vi "S4GUI.vi"() -> ()   [LabVIEW 2018] (continued)
            n2040 = call-dynamic "Write Suffix.vi"("error in (no error)"=w4728, "Suffix"=w4747, "Interface in"=w4729) -> ("error out"=w4746:errorcluster, "Interface out"=w4740:refnum<class "Interface.lvclass">)  [unwired: 7 in]
            n2041 = call-dynamic "Write ObsType.vi"("error in (no error)"=w4746, "ObsType"=w4732, "Interface in"=w4740) -> ("error out"=w4745:errorcluster, "Interface out"=w4739:refnum<class "Interface.lvclass">)  [unwired: 7 in]
            n2042 = call-dynamic "Write Object.vi"("error in (no error)"=w4745, "Object"=w4731, "Interface in"=w4739) -> ("error out"=w4744:errorcluster, "Interface out"=w4738:refnum<class "Interface.lvclass">)  [unwired: 7 in]
            n2043 = call-dynamic "Write Comments.vi"("error in (no error)"=w4744, "Comments"=w4733, "Interface in"=w4738) -> ("error out"=w4727:errorcluster, "Interface out"=w4726:refnum<class "Interface.lvclass">)  [unwired: 7 in]
            n2044 = call-dynamic "Write Observer.vi"("error in (no error)"=w4727, "Observer"=w4730, "Interface in"=w4726) -> ("error out"=w4722:errorcluster, "Interface out"=w4721:refnum<class "Interface.lvclass">)  [unwired: 7 in]
            n2045 = call-dynamic "Write Interface.vi"("error in (no error)"=w4722, "Interface.lvclass"=w4721, "Channel in"=w4741) -> ("error out"=w4717:errorcluster, "Channel out"=w4720:refnum<class "Channel.lvclass">)  [unwired: 7 in]
            n2046 = call-dynamic "Read State Machine.vi"("error in (no error)"=w4717, "Device in"=w4720) -> ("error out"=w4725:errorcluster, "State Machine.lvclass"=w4715:refnum<class "State Machine.lvclass">, "Device out"=w4719:refnum<class "Channel.lvclass">)  [unwired: 7 in]
            n2047 = call "Next State.vi"("error in (no error)"=w4725, "New_State"=12, "State Machine in"=w4715) -> ("error out"=w4724:errorcluster, "State Machine out"=w4714:refnum<class "State Machine.lvclass">)  [unwired: 7 in]
            n2048 = call-dynamic "Write State Machine.vi"("error in (no error)"=w4724, "State Machine.lvclass"=w4714, "Device in"=w4719) -> ("error out"=w4716:errorcluster, "Device out"=w4718:refnum<class "Channel.lvclass">)  [unwired: 7 in]
            n2049 = call-dynamic "Write Channel.vi"("error in (no error)"=w4716, "Channel.lvclass"=w4718, "Acquisition in"=w4736) -> ("error out"=w4734:errorcluster, "Acquisition out"=w4735:refnum<class "Acquisition.lvclass">)  [unwired: 7 in]
            n2050 = call-dynamic "Write AcquisitionD.vi"("error in (no error)"=w4734, "Acquisition.lvclass"=w4735, "S4ACS_GUI in"=w4737) -> ("error out"=w4748:errorcluster, "S4ACS_GUI out"=w4749:refnum<class "S4GUI.lvclass">)  [unwired: 7 in]
          }
        }
      }
      event "object suffix", "dflat suffix", "sflat suffix", "dark suffix", "zero suffix", "focus suffix": Value Change {
        # "Remove todos <\\n> e <space> do sufixo:"
        n2051 = event-data() -> ("NewVal"=w4760:string)  [unwired: 1 in, 5 out]
        n2052 = To Lower Case(string=w4760) -> (all lower case string=w4759:string)
        n2053 = call <vilib>:"Trim Whitespace.vi"("string"=w4759) -> ("trimmed string"=w4758:string)  [unwired: 1 in]
        n2054 = Search and Replace String(replace all?=TRUE ("replace all? (F)"), input string=w4758, search string="\n") -> (result string=w4756:string)  [unwired: 5 in, 3 out]
        n2055 = call <vilib>:"Space Constant.vi"() -> ("String"=w4754:string)
        n2056 = Search and Replace String(replace all?=TRUE ("replace all? (F)"), input string=w4756, search string=w4754) -> (result string=w4757:string)  [unwired: 5 in, 3 out]
        n2057 = stacked-sequence {
          seq-local: [w4796 _ _ _] -> [_ w4854 _ _]
          seq-local: [w4795 _ _ _] -> [_ w4853 _ _]
          seq-local: [_ w4852 _ _] -> [_ _ w4897 _]
          seq-local: [_ w4851 _ _] -> [_ _ w4896 _]
          seq-local: [_ _ w4895 _] -> [_ _ _ w4940]
          seq-local: [_ _ w4894 _] -> [_ _ _ w4939]
          tunnel: w4767 -> [w4808 _ _ _]
          tunnel: w4768 -> [w4807 _ _ _]
          tunnel: [_ _ _ w4938] -> w4762
          tunnel: [_ _ _ w4937] -> w4761
          tunnel: w4757 -> [w4794 w4850 w4893 w4936]
          tunnel: w4765 -> [w4793 w4849 w4879 w4922]
          tunnel: w4763 -> [w4792 w4835 w4878 w4921]
          tunnel: w4766 -> [w4791 w4834 w4877 w4920]
          tunnel: w4764 -> [w4790 w4833 w4876 w4919]
          frame #0 {
            # "observer"
            # "comment"
            # "object"
            # "suffix"
            # "obsType"
            n2058 = call-dynamic "Read AcquisitionA.vi"("error in (no error)"=w4808, "S4ACS_GUI in"=w4807) -> ("error out"=w4806:errorcluster, "Acquisition.lvclass"=w4805:refnum<class "Acquisition.lvclass">, "S4ACS_GUI out"=w4800:refnum<class "S4GUI.lvclass">)  [unwired: 7 in]
            n2059 = call-dynamic "Read Channel.vi"("error in (no error)"=w4806, "Acquisition in"=w4805) -> ("error out"=w4770:errorcluster, "Channel.lvclass"=w4773:refnum<class "Channel.lvclass">, "Acquisition out"=w4799:refnum<class "Acquisition.lvclass">)  [unwired: 7 in]
            n2060 = local read "Filter1"() -> (w4771:u8)
            n2061 = call-dynamic "Write Filter.vi"("error in (no error)"=w4770, "Filter"=w4771, "Channel in"=w4773) -> ("error out"=w4769:errorcluster, "Channel out"=w4772:refnum<class "Channel.lvclass">)  [unwired: 7 in]
            n2062 = call-dynamic "Read Interface.vi"("error in (no error)"=w4769, "Channel in"=w4772) -> ("error out"=w4786:errorcluster, "Interface.lvclass"=w4787:refnum<class "Interface.lvclass">, "Channel out"=w4804:refnum<class "Channel.lvclass">)  [unwired: 7 in]
            n2063 = call-dynamic "Write Suffix.vi"("error in (no error)"=w4786, "Suffix"=w4794, "Interface in"=w4787) -> ("error out"=w4811:errorcluster, "Interface out"=w4803:refnum<class "Interface.lvclass">)  [unwired: 7 in]
            n2064 = call-dynamic "Write ObsType.vi"("error in (no error)"=w4811, "ObsType"=w4792, "Interface in"=w4803) -> ("error out"=w4810:errorcluster, "Interface out"=w4802:refnum<class "Interface.lvclass">)  [unwired: 7 in]
            n2065 = call-dynamic "Write Object.vi"("error in (no error)"=w4810, "Object"=w4791, "Interface in"=w4802) -> ("error out"=w4809:errorcluster, "Interface out"=w4801:refnum<class "Interface.lvclass">)  [unwired: 7 in]
            n2066 = call-dynamic "Write Comments.vi"("error in (no error)"=w4809, "Comments"=w4793, "Interface in"=w4801) -> ("error out"=w4789:errorcluster, "Interface out"=w4788:refnum<class "Interface.lvclass">)  [unwired: 7 in]
            n2067 = call-dynamic "Write Observer.vi"("error in (no error)"=w4789, "Observer"=w4790, "Interface in"=w4788) -> ("error out"=w4784:errorcluster, "Interface out"=w4785:refnum<class "Interface.lvclass">)  [unwired: 7 in]
            n2068 = call-dynamic "Write Interface.vi"("error in (no error)"=w4784, "Interface.lvclass"=w4785, "Channel in"=w4804) -> ("error out"=w4780:errorcluster, "Channel out"=w4783:refnum<class "Channel.lvclass">)  [unwired: 7 in]
            n2069 = call-dynamic "Read State Machine.vi"("error in (no error)"=w4780, "Device in"=w4783) -> ("error out"=w4779:errorcluster, "State Machine.lvclass"=w4777:refnum<class "State Machine.lvclass">, "Device out"=w4782:refnum<class "Channel.lvclass">)  [unwired: 7 in]
            n2070 = call "Next State.vi"("error in (no error)"=w4779, "New_State"=12, "State Machine in"=w4777) -> ("error out"=w4778:errorcluster, "State Machine out"=w4776:refnum<class "State Machine.lvclass">)  [unwired: 7 in]
            n2071 = call-dynamic "Write State Machine.vi"("error in (no error)"=w4778, "State Machine.lvclass"=w4776, "Device in"=w4782) -> ("error out"=w4775:errorcluster, "Device out"=w4781:refnum<class "Channel.lvclass">)  [unwired: 7 in]
            n2072 = call-dynamic "Write Channel.vi"("error in (no error)"=w4775, "Channel.lvclass"=w4781, "Acquisition in"=w4799) -> ("error out"=w4797:errorcluster, "Acquisition out"=w4798:refnum<class "Acquisition.lvclass">)  [unwired: 7 in]
            n2073 = call-dynamic "Write AcquisitionA.vi"("error in (no error)"=w4797, "Acquisition.lvclass"=w4798, "S4ACS_GUI in"=w4800) -> ("error out"=w4795:errorcluster, "S4ACS_GUI out"=w4796:refnum<class "S4GUI.lvclass">)  [unwired: 7 in]
          }
          frame #1 {
            # "object"
            # "suffix"
            # "obsType"
            n2074 = call "Read AcquisitionB.vi"("error in (no error)"=w4853, "S4ACS_GUI in"=w4854) -> ("error out"=w4839:errorcluster, "Acquisition.lvclass"=w4840:refnum<class "Acquisition.lvclass">, "S4ACS_GUI out"=w4845:refnum<class "S4GUI.lvclass">)  [unwired: 7 in]
            n2075 = call-dynamic "Read Channel.vi"("error in (no error)"=w4839, "Acquisition in"=w4840) -> ("error out"=w4813:errorcluster, "Channel.lvclass"=w4815:refnum<class "Channel.lvclass">, "Acquisition out"=w4846:refnum<class "Acquisition.lvclass">)  [unwired: 7 in]
            n2076 = local read "Filter2"() -> (w4816:u8)
            n2077 = call-dynamic "Write Filter.vi"("error in (no error)"=w4813, "Filter"=w4816, "Channel in"=w4815) -> ("error out"=w4812:errorcluster, "Channel out"=w4814:refnum<class "Channel.lvclass">)  [unwired: 7 in]
            n2078 = call-dynamic "Read Interface.vi"("error in (no error)"=w4812, "Channel in"=w4814) -> ("error out"=w4827:errorcluster, "Interface.lvclass"=w4828:refnum<class "Interface.lvclass">, "Channel out"=w4841:refnum<class "Channel.lvclass">)  [unwired: 7 in]
            n2079 = call-dynamic "Write Suffix.vi"("error in (no error)"=w4827, "Suffix"=w4850, "Interface in"=w4828) -> ("error out"=w4836:errorcluster, "Interface out"=w4842:refnum<class "Interface.lvclass">)  [unwired: 7 in]
            n2080 = call-dynamic "Write ObsType.vi"("error in (no error)"=w4836, "ObsType"=w4835, "Interface in"=w4842) -> ("error out"=w4837:errorcluster, "Interface out"=w4843:refnum<class "Interface.lvclass">)  [unwired: 7 in]
            n2081 = call-dynamic "Write Object.vi"("error in (no error)"=w4837, "Object"=w4834, "Interface in"=w4843) -> ("error out"=w4838:errorcluster, "Interface out"=w4844:refnum<class "Interface.lvclass">)  [unwired: 7 in]
            n2082 = call-dynamic "Write Comments.vi"("error in (no error)"=w4838, "Comments"=w4849, "Interface in"=w4844) -> ("error out"=w4830:errorcluster, "Interface out"=w4829:refnum<class "Interface.lvclass">)  [unwired: 7 in]
            n2083 = call-dynamic "Write Observer.vi"("error in (no error)"=w4830, "Observer"=w4833, "Interface in"=w4829) -> ("error out"=w4831:errorcluster, "Interface out"=w4832:refnum<class "Interface.lvclass">)  [unwired: 7 in]
            n2084 = call-dynamic "Write Interface.vi"("error in (no error)"=w4831, "Interface.lvclass"=w4832, "Channel in"=w4841) -> ("error out"=w4820:errorcluster, "Channel out"=w4821:refnum<class "Channel.lvclass">)  [unwired: 7 in]
            n2085 = call-dynamic "Read State Machine.vi"("error in (no error)"=w4820, "Device in"=w4821) -> ("error out"=w4826:errorcluster, "State Machine.lvclass"=w4824:refnum<class "State Machine.lvclass">, "Device out"=w4819:refnum<class "Channel.lvclass">)  [unwired: 7 in]
            n2086 = call "Next State.vi"("error in (no error)"=w4826, "New_State"=12, "State Machine in"=w4824) -> ("error out"=w4825:errorcluster, "State Machine out"=w4823:refnum<class "State Machine.lvclass">)  [unwired: 7 in]
            n2087 = call-dynamic "Write State Machine.vi"("error in (no error)"=w4825, "State Machine.lvclass"=w4823, "Device in"=w4819) -> ("error out"=w4817:errorcluster, "Device out"=w4818:refnum<class "Channel.lvclass">)  [unwired: 7 in]
            n2088 = call-dynamic "Write Channel.vi"("error in (no error)"=w4817, "Channel.lvclass"=w4818, "Acquisition in"=w4846) -> ("error out"=w4848:errorcluster, "Acquisition out"=w4847:refnum<class "Acquisition.lvclass">)  [unwired: 7 in]
            n2089 = call "Write AcquisitionB.vi"("error in (no error)"=w4848, "Acquisition.lvclass"=w4847, "S4ACS_GUI in"=w4845) -> ("error out"=w4851:errorcluster, "S4ACS_GUI out"=w4852:refnum<class "S4GUI.lvclass">)  [unwired: 7 in]
          }
          frame #2 {
            # "object"
            # "suffix"
            # "obsType"
            n2090 = call-dynamic "Read AcquisitionC.vi"("error in (no error)"=w4896, "S4ACS_GUI in"=w4897) -> ("error out"=w4889:errorcluster, "Acquisition.lvclass"=w4888:refnum<class "Acquisition.lvclass">, "S4ACS_GUI out"=w4883:refnum<class "S4GUI.lvclass">)  [unwired: 7 in]
            n2091 = call-dynamic "Read Channel.vi"("error in (no error)"=w4889, "Acquisition in"=w4888) -> ("error out"=w4856:errorcluster, "Channel.lvclass"=w4858:refnum<class "Channel.lvclass">, "Acquisition out"=w4882:refnum<class "Acquisition.lvclass">)  [unwired: 7 in]
            n2092 = local read "Filter3"() -> (w4859:u8)
            n2093 = call-dynamic "Write Filter.vi"("error in (no error)"=w4856, "Filter"=w4859, "Channel in"=w4858) -> ("error out"=w4855:errorcluster, "Channel out"=w4857:refnum<class "Channel.lvclass">)  [unwired: 7 in]
            n2094 = call-dynamic "Read Interface.vi"("error in (no error)"=w4855, "Channel in"=w4857) -> ("error out"=w4874:errorcluster, "Interface.lvclass"=w4875:refnum<class "Interface.lvclass">, "Channel out"=w4887:refnum<class "Channel.lvclass">)  [unwired: 7 in]
            n2095 = call-dynamic "Write Suffix.vi"("error in (no error)"=w4874, "Suffix"=w4893, "Interface in"=w4875) -> ("error out"=w4892:errorcluster, "Interface out"=w4886:refnum<class "Interface.lvclass">)  [unwired: 7 in]
            n2096 = call-dynamic "Write ObsType.vi"("error in (no error)"=w4892, "ObsType"=w4878, "Interface in"=w4886) -> ("error out"=w4891:errorcluster, "Interface out"=w4885:refnum<class "Interface.lvclass">)  [unwired: 7 in]
            n2097 = call-dynamic "Write Object.vi"("error in (no error)"=w4891, "Object"=w4877, "Interface in"=w4885) -> ("error out"=w4890:errorcluster, "Interface out"=w4884:refnum<class "Interface.lvclass">)  [unwired: 7 in]
            n2098 = call-dynamic "Write Comments.vi"("error in (no error)"=w4890, "Comments"=w4879, "Interface in"=w4884) -> ("error out"=w4871:errorcluster, "Interface out"=w4870:refnum<class "Interface.lvclass">)  [unwired: 7 in]
            n2099 = call-dynamic "Write Observer.vi"("error in (no error)"=w4871, "Observer"=w4876, "Interface in"=w4870) -> ("error out"=w4872:errorcluster, "Interface out"=w4873:refnum<class "Interface.lvclass">)  [unwired: 7 in]
            n2100 = call-dynamic "Write Interface.vi"("error in (no error)"=w4872, "Interface.lvclass"=w4873, "Channel in"=w4887) -> ("error out"=w4865:errorcluster, "Channel out"=w4866:refnum<class "Channel.lvclass">)  [unwired: 7 in]
            n2101 = call-dynamic "Read State Machine.vi"("error in (no error)"=w4865, "Device in"=w4866) -> ("error out"=w4869:errorcluster, "State Machine.lvclass"=w4862:refnum<class "State Machine.lvclass">, "Device out"=w4864:refnum<class "Channel.lvclass">)  [unwired: 7 in]
            n2102 = call "Next State.vi"("error in (no error)"=w4869, "New_State"=12, "State Machine in"=w4862) -> ("error out"=w4868:errorcluster, "State Machine out"=w4861:refnum<class "State Machine.lvclass">)  [unwired: 7 in]
            n2103 = call-dynamic "Write State Machine.vi"("error in (no error)"=w4868, "State Machine.lvclass"=w4861, "Device in"=w4864) -> ("error out"=w4860:errorcluster, "Device out"=w4863:refnum<class "Channel.lvclass">)  [unwired: 7 in]
            n2104 = call-dynamic "Write Channel.vi"("error in (no error)"=w4860, "Channel.lvclass"=w4863, "Acquisition in"=w4882) -> ("error out"=w4880:errorcluster, "Acquisition out"=w4881:refnum<class "Acquisition.lvclass">)  [unwired: 7 in]
            n2105 = call-dynamic "Write AcquisitionC.vi"("error in (no error)"=w4880, "Acquisition.lvclass"=w4881, "S4ACS_GUI in"=w4883) -> ("error out"=w4894:errorcluster, "S4ACS_GUI out"=w4895:refnum<class "S4GUI.lvclass">)  [unwired: 7 in]
          }
          frame #3 {
            # "object"
            # "suffix"
            # "obsType"
            n2106 = call-dynamic "Read AcquisitionD.vi"("error in (no error)"=w4939, "S4ACS_GUI in"=w4940) -> ("error out"=w4932:errorcluster, "Acquisition.lvclass"=w4931:refnum<class "Acquisition.lvclass">, "S4ACS_GUI out"=w4926:refnum<class "S4GUI.lvclass">)  [unwired: 7 in]
            n2107 = call-dynamic "Read Channel.vi"("error in (no error)"=w4932, "Acquisition in"=w4931) -> ("error out"=w4899:errorcluster, "Channel.lvclass"=w4901:refnum<class "Channel.lvclass">, "Acquisition out"=w4925:refnum<class "Acquisition.lvclass">)  [unwired: 7 in]
            n2108 = local read "Filter4"() -> (w4902:u8)
            n2109 = call-dynamic "Write Filter.vi"("error in (no error)"=w4899, "Filter"=w4902, "Channel in"=w4901) -> ("error out"=w4898:errorcluster, "Channel out"=w4900:refnum<class "Channel.lvclass">)  [unwired: 7 in]
            n2110 = call-dynamic "Read Interface.vi"("error in (no error)"=w4898, "Channel in"=w4900) -> ("error out"=w4917:errorcluster, "Interface.lvclass"=w4918:refnum<class "Interface.lvclass">, "Channel out"=w4930:refnum<class "Channel.lvclass">)  [unwired: 7 in]
            n2111 = call-dynamic "Write Suffix.vi"("error in (no error)"=w4917, "Suffix"=w4936, "Interface in"=w4918) -> ("error out"=w4935:errorcluster, "Interface out"=w4929:refnum<class "Interface.lvclass">)  [unwired: 7 in]
            n2112 = call-dynamic "Write ObsType.vi"("error in (no error)"=w4935, "ObsType"=w4921, "Interface in"=w4929) -> ("error out"=w4934:errorcluster, "Interface out"=w4928:refnum<class "Interface.lvclass">)  [unwired: 7 in]
            n2113 = call-dynamic "Write Object.vi"("error in (no error)"=w4934, "Object"=w4920, "Interface in"=w4928) -> ("error out"=w4933:errorcluster, "Interface out"=w4927:refnum<class "Interface.lvclass">)  [unwired: 7 in]
            n2114 = call-dynamic "Write Comments.vi"("error in (no error)"=w4933, "Comments"=w4922, "Interface in"=w4927) -> ("error out"=w4916:errorcluster, "Interface out"=w4915:refnum<class "Interface.lvclass">)  [unwired: 7 in]
            n2115 = call-dynamic "Write Observer.vi"("error in (no error)"=w4916, "Observer"=w4919, "Interface in"=w4915) -> ("error out"=w4911:errorcluster, "Interface out"=w4910:refnum<class "Interface.lvclass">)  [unwired: 7 in]
            n2116 = call-dynamic "Write Interface.vi"("error in (no error)"=w4911, "Interface.lvclass"=w4910, "Channel in"=w4930) -> ("error out"=w4906:errorcluster, "Channel out"=w4909:refnum<class "Channel.lvclass">)  [unwired: 7 in]
            n2117 = call-dynamic "Read State Machine.vi"("error in (no error)"=w4906, "Device in"=w4909) -> ("error out"=w4914:errorcluster, "State Machine.lvclass"=w4904:refnum<class "State Machine.lvclass">, "Device out"=w4908:refnum<class "Channel.lvclass">)  [unwired: 7 in]
            n2118 = call "Next State.vi"("error in (no error)"=w4914, "New_State"=12, "State Machine in"=w4904) -> ("error out"=w4913:errorcluster, "State Machine out"=w4903:refnum<class "State Machine.lvclass">)  [unwired: 7 in]
            n2119 = call-dynamic "Write State Machine.vi"("error in (no error)"=w4913, "State Machine.lvclass"=w4903, "Device in"=w4908) -> ("error out"=w4905:errorcluster, "Device out"=w4907:refnum<class "Channel.lvclass">)  [unwired: 7 in]
            n2120 = call-dynamic "Write Channel.vi"("error in (no error)"=w4905, "Channel.lvclass"=w4907, "Acquisition in"=w4925) -> ("error out"=w4923:errorcluster, "Acquisition out"=w4924:refnum<class "Acquisition.lvclass">)  [unwired: 7 in]
            n2121 = call-dynamic "Write AcquisitionD.vi"("error in (no error)"=w4923, "Acquisition.lvclass"=w4924, "S4ACS_GUI in"=w4926) -> ("error out"=w4937:errorcluster, "S4ACS_GUI out"=w4938:refnum<class "S4GUI.lvclass">)  [unwired: 7 in]
          }
        }
      }
      event "Observer": Value Change {
        n2122 = event-data() -> ("NewVal"=w4941:string)  [unwired: 1 in, 5 out]
        n2123 = disable-structure shown="Enabled" {
          disable-tunnel: w4944 -> [w4959 w4960]
          disable-tunnel: w4941 -> [w4958 _]
          disable-tunnel: [w4957 w4960] -> w4943
          frame Disabled {
            n2124 = String Length(string=w4958) -> (length=w4956:i32)
            n2125 = Equal To 0?(x=w4956) -> (x = 0?=w4955:bool)
            n2126 = Select(t=u32 16777216, s=w4955, f=u32 16777225) -> (s? t:f=w4953:u32)
            n2127 = property on="Observer" class="Str"(error in=w4959, "Text.BGColor"=w4953) -> (error out=w4957:errorcluster)  [unwired: 1 in, 1 out]
          }
          frame Enabled {
            # "Não se usa mais o texto de fundo\ndo controle \"Observer\""
          }
        }
        n2128 = case shown="False" FALSE {
          tunnel: w4951 -> [w4969 w5143]
          tunnel: w4950 -> [w4968 _]
          tunnel: w4949 -> [w4967 _]
          tunnel: w4948 -> [w4966 _]
          tunnel: w4941 -> [w4965 _]
          tunnel: w4947 -> [w4964 _]
          tunnel: [w4963 w5143] -> w4946
          tunnel: [w4962 w5142] -> w4945
          tunnel: w4943 -> [w4961 w5142]
          frame False {
            n2129 = stacked-sequence {
              seq-local: [w4997 _ _ _] -> [_ w5055 _ _]
              seq-local: [w4996 _ _ _] -> [_ w5054 _ _]
              seq-local: [_ w5053 _ _] -> [_ _ w5098 _]
              seq-local: [_ w5052 _ _] -> [_ _ w5097 _]
              seq-local: [_ _ w5096 _] -> [_ _ _ w5141]
              seq-local: [_ _ w5095 _] -> [_ _ _ w5140]
              tunnel: w4961 -> [w5009 _ _ _]
              tunnel: w4969 -> [w5008 _ _ _]
              tunnel: [_ _ _ w5139] -> w4963
              tunnel: [_ _ _ w5138] -> w4962
              tunnel: w4967 -> [w4995 w5051 w5094 w5137]
              tunnel: w4966 -> [w4994 w5050 w5080 w5123]
              tunnel: w4964 -> [w4993 w5036 w5079 w5122]
              tunnel: w4968 -> [w4992 w5035 w5078 w5121]
              tunnel: w4965 -> [w4991 w5034 w5077 w5120]
              frame #0 {
                # "observer"
                # "comment"
                # "object"
                # "suffix"
                # "obsType"
                n2130 = call-dynamic "Read AcquisitionA.vi"("error in (no error)"=w5009, "S4ACS_GUI in"=w5008) -> ("error out"=w5007:errorcluster, "Acquisition.lvclass"=w5006:refnum<class "Acquisition.lvclass">, "S4ACS_GUI out"=w5001:refnum<class "S4GUI.lvclass">)  [unwired: 7 in]
                n2131 = call-dynamic "Read Channel.vi"("error in (no error)"=w5007, "Acquisition in"=w5006) -> ("error out"=w4971:errorcluster, "Channel.lvclass"=w4974:refnum<class "Channel.lvclass">, "Acquisition out"=w5000:refnum<class "Acquisition.lvclass">)  [unwired: 7 in]
                n2132 = local read "Filter1"() -> (w4972:u8)
                n2133 = call-dynamic "Write Filter.vi"("error in (no error)"=w4971, "Filter"=w4972, "Channel in"=w4974) -> ("error out"=w4970:errorcluster, "Channel out"=w4973:refnum<class "Channel.lvclass">)  [unwired: 7 in]
                n2134 = call-dynamic "Read Interface.vi"("error in (no error)"=w4970, "Channel in"=w4973) -> ("error out"=w4987:errorcluster, "Interface.lvclass"=w4988:refnum<class "Interface.lvclass">, "Channel out"=w5005:refnum<class "Channel.lvclass">)  [unwired: 7 in]
                n2135 = call-dynamic "Write Suffix.vi"("error in (no error)"=w4987, "Suffix"=w4995, "Interface in"=w4988) -> ("error out"=w5012:errorcluster, "Interface out"=w5004:refnum<class "Interface.lvclass">)  [unwired: 7 in]
                n2136 = call-dynamic "Write ObsType.vi"("error in (no error)"=w5012, "ObsType"=w4993, "Interface in"=w5004) -> ("error out"=w5011:errorcluster, "Interface out"=w5003:refnum<class "Interface.lvclass">)  [unwired: 7 in]
                n2137 = call-dynamic "Write Object.vi"("error in (no error)"=w5011, "Object"=w4992, "Interface in"=w5003) -> ("error out"=w5010:errorcluster, "Interface out"=w5002:refnum<class "Interface.lvclass">)  [unwired: 7 in]
                n2138 = call-dynamic "Write Comments.vi"("error in (no error)"=w5010, "Comments"=w4994, "Interface in"=w5002) -> ("error out"=w4990:errorcluster, "Interface out"=w4989:refnum<class "Interface.lvclass">)  [unwired: 7 in]
                n2139 = call-dynamic "Write Observer.vi"("error in (no error)"=w4990, "Observer"=w4991, "Interface in"=w4989) -> ("error out"=w4985:errorcluster, "Interface out"=w4986:refnum<class "Interface.lvclass">)  [unwired: 7 in]
                n2140 = call-dynamic "Write Interface.vi"("error in (no error)"=w4985, "Interface.lvclass"=w4986, "Channel in"=w5005) -> ("error out"=w4981:errorcluster, "Channel out"=w4984:refnum<class "Channel.lvclass">)  [unwired: 7 in]
                n2141 = call-dynamic "Read State Machine.vi"("error in (no error)"=w4981, "Device in"=w4984) -> ("error out"=w4980:errorcluster, "State Machine.lvclass"=w4978:refnum<class "State Machine.lvclass">, "Device out"=w4983:refnum<class "Channel.lvclass">)  [unwired: 7 in]
                n2142 = call "Next State.vi"("error in (no error)"=w4980, "New_State"=12, "State Machine in"=w4978) -> ("error out"=w4979:errorcluster, "State Machine out"=w4977:refnum<class "State Machine.lvclass">)  [unwired: 7 in]
                n2143 = call-dynamic "Write State Machine.vi"("error in (no error)"=w4979, "State Machine.lvclass"=w4977, "Device in"=w4983) -> ("error out"=w4976:errorcluster, "Device out"=w4982:refnum<class "Channel.lvclass">)  [unwired: 7 in]
                n2144 = call-dynamic "Write Channel.vi"("error in (no error)"=w4976, "Channel.lvclass"=w4982, "Acquisition in"=w5000) -> ("error out"=w4998:errorcluster, "Acquisition out"=w4999:refnum<class "Acquisition.lvclass">)  [unwired: 7 in]
                n2145 = call-dynamic "Write AcquisitionA.vi"("error in (no error)"=w4998, "Acquisition.lvclass"=w4999, "S4ACS_GUI in"=w5001) -> ("error out"=w4996:errorcluster, "S4ACS_GUI out"=w4997:refnum<class "S4GUI.lvclass">)  [unwired: 7 in]
              }
              frame #1 {
                # "object"
                # "suffix"
                # "obsType"
                n2146 = call "Read AcquisitionB.vi"("error in (no error)"=w5054, "S4ACS_GUI in"=w5055) -> ("error out"=w5040:errorcluster, "Acquisition.lvclass"=w5041:refnum<class "Acquisition.lvclass">, "S4ACS_GUI out"=w5046:refnum<class "S4GUI.lvclass">)  [unwired: 7 in]
                n2147 = call-dynamic "Read Channel.vi"("error in (no error)"=w5040, "Acquisition in"=w5041) -> ("error out"=w5014:errorcluster, "Channel.lvclass"=w5016:refnum<class "Channel.lvclass">, "Acquisition out"=w5047:refnum<class "Acquisition.lvclass">)  [unwired: 7 in]
                n2148 = local read "Filter2"() -> (w5017:u8)
                n2149 = call-dynamic "Write Filter.vi"("error in (no error)"=w5014, "Filter"=w5017, "Channel in"=w5016) -> ("error out"=w5013:errorcluster, "Channel out"=w5015:refnum<class "Channel.lvclass">)  [unwired: 7 in]
                n2150 = call-dynamic "Read Interface.vi"("error in (no error)"=w5013, "Channel in"=w5015) -> ("error out"=w5028:errorcluster, "Interface.lvclass"=w5029:refnum<class "Interface.lvclass">, "Channel out"=w5042:refnum<class "Channel.lvclass">)  [unwired: 7 in]
                n2151 = call-dynamic "Write Suffix.vi"("error in (no error)"=w5028, "Suffix"=w5051, "Interface in"=w5029) -> ("error out"=w5037:errorcluster, "Interface out"=w5043:refnum<class "Interface.lvclass">)  [unwired: 7 in]
                n2152 = call-dynamic "Write ObsType.vi"("error in (no error)"=w5037, "ObsType"=w5036, "Interface in"=w5043) -> ("error out"=w5038:errorcluster, "Interface out"=w5044:refnum<class "Interface.lvclass">)  [unwired: 7 in]
                n2153 = call-dynamic "Write Object.vi"("error in (no error)"=w5038, "Object"=w5035, "Interface in"=w5044) -> ("error out"=w5039:errorcluster, "Interface out"=w5045:refnum<class "Interface.lvclass">)  [unwired: 7 in]
                n2154 = call-dynamic "Write Comments.vi"("error in (no error)"=w5039, "Comments"=w5050, "Interface in"=w5045) -> ("error out"=w5031:errorcluster, "Interface out"=w5030:refnum<class "Interface.lvclass">)  [unwired: 7 in]
                n2155 = call-dynamic "Write Observer.vi"("error in (no error)"=w5031, "Observer"=w5034, "Interface in"=w5030) -> ("error out"=w5032:errorcluster, "Interface out"=w5033:refnum<class "Interface.lvclass">)  [unwired: 7 in]
                n2156 = call-dynamic "Write Interface.vi"("error in (no error)"=w5032, "Interface.lvclass"=w5033, "Channel in"=w5042) -> ("error out"=w5021:errorcluster, "Channel out"=w5022:refnum<class "Channel.lvclass">)  [unwired: 7 in]
                n2157 = call-dynamic "Read State Machine.vi"("error in (no error)"=w5021, "Device in"=w5022) -> ("error out"=w5027:errorcluster, "State Machine.lvclass"=w5025:refnum<class "State Machine.lvclass">, "Device out"=w5020:refnum<class "Channel.lvclass">)  [unwired: 7 in]
                n2158 = call "Next State.vi"("error in (no error)"=w5027, "New_State"=12, "State Machine in"=w5025) -> ("error out"=w5026:errorcluster, "State Machine out"=w5024:refnum<class "State Machine.lvclass">)  [unwired: 7 in]
                n2159 = call-dynamic "Write State Machine.vi"("error in (no error)"=w5026, "State Machine.lvclass"=w5024, "Device in"=w5020) -> ("error out"=w5018:errorcluster, "Device out"=w5019:refnum<class "Channel.lvclass">)  [unwired: 7 in]
                n2160 = call-dynamic "Write Channel.vi"("error in (no error)"=w5018, "Channel.lvclass"=w5019, "Acquisition in"=w5047) -> ("error out"=w5049:errorcluster, "Acquisition out"=w5048:refnum<class "Acquisition.lvclass">)  [unwired: 7 in]
                n2161 = call "Write AcquisitionB.vi"("error in (no error)"=w5049, "Acquisition.lvclass"=w5048, "S4ACS_GUI in"=w5046) -> ("error out"=w5052:errorcluster, "S4ACS_GUI out"=w5053:refnum<class "S4GUI.lvclass">)  [unwired: 7 in]
              }
              frame #2 {
                # "object"
                # "suffix"
                # "obsType"
                n2162 = call-dynamic "Read AcquisitionC.vi"("error in (no error)"=w5097, "S4ACS_GUI in"=w5098) -> ("error out"=w5090:errorcluster, "Acquisition.lvclass"=w5089:refnum<class "Acquisition.lvclass">, "S4ACS_GUI out"=w5084:refnum<class "S4GUI.lvclass">)  [unwired: 7 in]
                n2163 = call-dynamic "Read Channel.vi"("error in (no error)"=w5090, "Acquisition in"=w5089) -> ("error out"=w5057:errorcluster, "Channel.lvclass"=w5059:refnum<class "Channel.lvclass">, "Acquisition out"=w5083:refnum<class "Acquisition.lvclass">)  [unwired: 7 in]
                n2164 = local read "Filter3"() -> (w5060:u8)
                n2165 = call-dynamic "Write Filter.vi"("error in (no error)"=w5057, "Filter"=w5060, "Channel in"=w5059) -> ("error out"=w5056:errorcluster, "Channel out"=w5058:refnum<class "Channel.lvclass">)  [unwired: 7 in]
                n2166 = call-dynamic "Read Interface.vi"("error in (no error)"=w5056, "Channel in"=w5058) -> ("error out"=w5075:errorcluster, "Interface.lvclass"=w5076:refnum<class "Interface.lvclass">, "Channel out"=w5088:refnum<class "Channel.lvclass">)  [unwired: 7 in]
                n2167 = call-dynamic "Write Suffix.vi"("error in (no error)"=w5075, "Suffix"=w5094, "Interface in"=w5076) -> ("error out"=w5093:errorcluster, "Interface out"=w5087:refnum<class "Interface.lvclass">)  [unwired: 7 in]
                n2168 = call-dynamic "Write ObsType.vi"("error in (no error)"=w5093, "ObsType"=w5079, "Interface in"=w5087) -> ("error out"=w5092:errorcluster, "Interface out"=w5086:refnum<class "Interface.lvclass">)  [unwired: 7 in]
                n2169 = call-dynamic "Write Object.vi"("error in (no error)"=w5092, "Object"=w5078, "Interface in"=w5086) -> ("error out"=w5091:errorcluster, "Interface out"=w5085:refnum<class "Interface.lvclass">)  [unwired: 7 in]
                n2170 = call-dynamic "Write Comments.vi"("error in (no error)"=w5091, "Comments"=w5080, "Interface in"=w5085) -> ("error out"=w5072:errorcluster, "Interface out"=w5071:refnum<class "Interface.lvclass">)  [unwired: 7 in]
                n2171 = call-dynamic "Write Observer.vi"("error in (no error)"=w5072, "Observer"=w5077, "Interface in"=w5071) -> ("error out"=w5073:errorcluster, "Interface out"=w5074:refnum<class "Interface.lvclass">)  [unwired: 7 in]
                n2172 = call-dynamic "Write Interface.vi"("error in (no error)"=w5073, "Interface.lvclass"=w5074, "Channel in"=w5088) -> ("error out"=w5066:errorcluster, "Channel out"=w5067:refnum<class "Channel.lvclass">)  [unwired: 7 in]
                n2173 = call-dynamic "Read State Machine.vi"("error in (no error)"=w5066, "Device in"=w5067) -> ("error out"=w5070:errorcluster, "State Machine.lvclass"=w5063:refnum<class "State Machine.lvclass">, "Device out"=w5065:refnum<class "Channel.lvclass">)  [unwired: 7 in]
                n2174 = call "Next State.vi"("error in (no error)"=w5070, "New_State"=12, "State Machine in"=w5063) -> ("error out"=w5069:errorcluster, "State Machine out"=w5062:refnum<class "State Machine.lvclass">)  [unwired: 7 in]
                n2175 = call-dynamic "Write State Machine.vi"("error in (no error)"=w5069, "State Machine.lvclass"=w5062, "Device in"=w5065) -> ("error out"=w5061:errorcluster, "Device out"=w5064:refnum<class "Channel.lvclass">)  [unwired: 7 in]
                n2176 = call-dynamic "Write Channel.vi"("error in (no error)"=w5061, "Channel.lvclass"=w5064, "Acquisition in"=w5083) -> ("error out"=w5081:errorcluster, "Acquisition out"=w5082:refnum<class "Acquisition.lvclass">)  [unwired: 7 in]
                n2177 = call-dynamic "Write AcquisitionC.vi"("error in (no error)"=w5081, "Acquisition.lvclass"=w5082, "S4ACS_GUI in"=w5084) -> ("error out"=w5095:errorcluster, "S4ACS_GUI out"=w5096:refnum<class "S4GUI.lvclass">)  [unwired: 7 in]
              }
              frame #3 {
                # "object"
                # "suffix"
                # "obsType"
                n2178 = call-dynamic "Read AcquisitionD.vi"("error in (no error)"=w5140, "S4ACS_GUI in"=w5141) -> ("error out"=w5133:errorcluster, "Acquisition.lvclass"=w5132:refnum<class "Acquisition.lvclass">, "S4ACS_GUI out"=w5127:refnum<class "S4GUI.lvclass">)  [unwired: 7 in]
                n2179 = call-dynamic "Read Channel.vi"("error in (no error)"=w5133, "Acquisition in"=w5132) -> ("error out"=w5100:errorcluster, "Channel.lvclass"=w5102:refnum<class "Channel.lvclass">, "Acquisition out"=w5126:refnum<class "Acquisition.lvclass">)  [unwired: 7 in]
                n2180 = local read "Filter4"() -> (w5103:u8)
                n2181 = call-dynamic "Write Filter.vi"("error in (no error)"=w5100, "Filter"=w5103, "Channel in"=w5102) -> ("error out"=w5099:errorcluster, "Channel out"=w5101:refnum<class "Channel.lvclass">)  [unwired: 7 in]
                n2182 = call-dynamic "Read Interface.vi"("error in (no error)"=w5099, "Channel in"=w5101) -> ("error out"=w5118:errorcluster, "Interface.lvclass"=w5119:refnum<class "Interface.lvclass">, "Channel out"=w5131:refnum<class "Channel.lvclass">)  [unwired: 7 in]
                n2183 = call-dynamic "Write Suffix.vi"("error in (no error)"=w5118, "Suffix"=w5137, "Interface in"=w5119) -> ("error out"=w5136:errorcluster, "Interface out"=w5130:refnum<class "Interface.lvclass">)  [unwired: 7 in]
                n2184 = call-dynamic "Write ObsType.vi"("error in (no error)"=w5136, "ObsType"=w5122, "Interface in"=w5130) -> ("error out"=w5135:errorcluster, "Interface out"=w5129:refnum<class "Interface.lvclass">)  [unwired: 7 in]
                n2185 = call-dynamic "Write Object.vi"("error in (no error)"=w5135, "Object"=w5121, "Interface in"=w5129) -> ("error out"=w5134:errorcluster, "Interface out"=w5128:refnum<class "Interface.lvclass">)  [unwired: 7 in]
                n2186 = call-dynamic "Write Comments.vi"("error in (no error)"=w5134, "Comments"=w5123, "Interface in"=w5128) -> ("error out"=w5117:errorcluster, "Interface out"=w5116:refnum<class "Interface.lvclass">)  [unwired: 7 in]
                n2187 = call-dynamic "Write Observer.vi"("error in (no error)"=w5117, "Observer"=w5120, "Interface in"=w5116) -> ("error out"=w5112:errorcluster, "Interface out"=w5111:refnum<class "Interface.lvclass">)  [unwired: 7 in]
                n2188 = call-dynamic "Write Interface.vi"("error in (no error)"=w5112, "Interface.lvclass"=w5111, "Channel in"=w5131) -> ("error out"=w5107:errorcluster, "Channel out"=w5110:refnum<class "Channel.lvclass">)  [unwired: 7 in]
                n2189 = call-dynamic "Read State Machine.vi"("error in (no error)"=w5107, "Device in"=w5110) -> ("error out"=w5115:errorcluster, "State Machine.lvclass"=w5105:refnum<class "State Machine.lvclass">, "Device out"=w5109:refnum<class "Channel.lvclass">)  [unwired: 7 in]
                n2190 = call "Next State.vi"("error in (no error)"=w5115, "New_State"=12, "State Machine in"=w5105) -> ("error out"=w5114:errorcluster, "State Machine out"=w5104:refnum<class "State Machine.lvclass">)  [unwired: 7 in]
                n2191 = call-dynamic "Write State Machine.vi"("error in (no error)"=w5114, "State Machine.lvclass"=w5104, "Device in"=w5109) -> ("error out"=w5106:errorcluster, "Device out"=w5108:refnum<class "Channel.lvclass">)  [unwired: 7 in]
                n2192 = call-dynamic "Write Channel.vi"("error in (no error)"=w5106, "Channel.lvclass"=w5108, "Acquisition in"=w5126) -> ("error out"=w5124:errorcluster, "Acquisition out"=w5125:refnum<class "Acquisition.lvclass">)  [unwired: 7 in]
                n2193 = call-dynamic "Write AcquisitionD.vi"("error in (no error)"=w5124, "Acquisition.lvclass"=w5125, "S4ACS_GUI in"=w5127) -> ("error out"=w5138:errorcluster, "S4ACS_GUI out"=w5139:refnum<class "S4GUI.lvclass">)  [unwired: 7 in]
              }
            }
          }
          frame True {
          }
        }
      }
      event "Observer": Mouse Enter {
        n2194 = event-data() -> ()  [unwired: 1 in, 4 out]
        n2195 = disable-structure shown="Enabled" {
          disable-tunnel: [w5149 w5152] -> w5145
          disable-tunnel: w5144 -> [w5147 w5152]
          frame Disabled {
            n2196 = property on="Observer" class="Str"() -> ("Value"=w5148:string)  [unwired: 2 in, 2 out]
            n2197 = String Length(string=w5148) -> (length=w5151:i32)
            n2198 = Equal To 0?(x=w5151) -> (x = 0?=w5150:bool)
            n2199 = property on="Observer" class="Str"(error in=w5147, "Caption.Visible"=w5150) -> (error out=w5149:errorcluster)  [unwired: 1 in, 1 out]
          }
          frame Enabled {
            # "Não se usa mais o texto de fundo\ndo controle \"Observer\""
          }
        }
      }
      event "set keywords": Value Change {
        n2200 = event-data() -> ()  [unwired: 1 in, 6 out]
      }
      event "Filter1", "Filter2", "Filter3", "Filter4": Value Change {
        n2201 = event-data() -> ()  [unwired: 1 in, 6 out]
        n2202 = stacked-sequence {
          seq-local: [w5191 _ _ _] -> [_ w5249 _ _]
          seq-local: [w5190 _ _ _] -> [_ w5248 _ _]
          seq-local: [_ w5247 _ _] -> [_ _ w5292 _]
          seq-local: [_ w5246 _ _] -> [_ _ w5291 _]
          seq-local: [_ _ w5290 _] -> [_ _ _ w5335]
          seq-local: [_ _ w5289 _] -> [_ _ _ w5334]
          tunnel: w5162 -> [w5203 _ _ _]
          tunnel: w5163 -> [w5202 _ _ _]
          tunnel: [_ _ _ w5333] -> w5156
          tunnel: [_ _ _ w5332] -> w5155
          tunnel: w5160 -> [w5189 w5245 w5288 w5331]
          tunnel: w5159 -> [w5188 w5244 w5274 w5317]
          tunnel: w5157 -> [w5187 w5230 w5273 w5316]
          tunnel: w5161 -> [w5186 w5229 w5272 w5315]
          tunnel: w5158 -> [w5185 w5228 w5271 w5314]
          frame #0 {
            # "observer"
            # "comment"
            # "object"
            # "suffix"
            # "obsType"
            n2203 = call-dynamic "Read AcquisitionA.vi"("error in (no error)"=w5203, "S4ACS_GUI in"=w5202) -> ("error out"=w5201:errorcluster, "Acquisition.lvclass"=w5200:refnum<class "Acquisition.lvclass">, "S4ACS_GUI out"=w5195:refnum<class "S4GUI.lvclass">)  [unwired: 7 in]
            n2204 = call-dynamic "Read Channel.vi"("error in (no error)"=w5201, "Acquisition in"=w5200) -> ("error out"=w5165:errorcluster, "Channel.lvclass"=w5168:refnum<class "Channel.lvclass">, "Acquisition out"=w5194:refnum<class "Acquisition.lvclass">)  [unwired: 7 in]
            n2205 = local read "Filter1"() -> (w5166:u8)
            n2206 = call-dynamic "Write Filter.vi"("error in (no error)"=w5165, "Filter"=w5166, "Channel in"=w5168) -> ("error out"=w5164:errorcluster, "Channel out"=w5167:refnum<class "Channel.lvclass">)  [unwired: 7 in]
            n2207 = call-dynamic "Read Interface.vi"("error in (no error)"=w5164, "Channel in"=w5167) -> ("error out"=w5181:errorcluster, "Interface.lvclass"=w5182:refnum<class "Interface.lvclass">, "Channel out"=w5199:refnum<class "Channel.lvclass">)  [unwired: 7 in]
            n2208 = call-dynamic "Write Suffix.vi"("error in (no error)"=w5181, "Suffix"=w5189, "Interface in"=w5182) -> ("error out"=w5206:errorcluster, "Interface out"=w5198:refnum<class "Interface.lvclass">)  [unwired: 7 in]
            n2209 = call-dynamic "Write ObsType.vi"("error in (no error)"=w5206, "ObsType"=w5187, "Interface in"=w5198) -> ("error out"=w5205:errorcluster, "Interface out"=w5197:refnum<class "Interface.lvclass">)  [unwired: 7 in]
            n2210 = call-dynamic "Write Object.vi"("error in (no error)"=w5205, "Object"=w5186, "Interface in"=w5197) -> ("error out"=w5204:errorcluster, "Interface out"=w5196:refnum<class "Interface.lvclass">)  [unwired: 7 in]
            n2211 = call-dynamic "Write Comments.vi"("error in (no error)"=w5204, "Comments"=w5188, "Interface in"=w5196) -> ("error out"=w5184:errorcluster, "Interface out"=w5183:refnum<class "Interface.lvclass">)  [unwired: 7 in]
            n2212 = call-dynamic "Write Observer.vi"("error in (no error)"=w5184, "Observer"=w5185, "Interface in"=w5183) -> ("error out"=w5179:errorcluster, "Interface out"=w5180:refnum<class "Interface.lvclass">)  [unwired: 7 in]
            n2213 = call-dynamic "Write Interface.vi"("error in (no error)"=w5179, "Interface.lvclass"=w5180, "Channel in"=w5199) -> ("error out"=w5175:errorcluster, "Channel out"=w5178:refnum<class "Channel.lvclass">)  [unwired: 7 in]
            n2214 = call-dynamic "Read State Machine.vi"("error in (no error)"=w5175, "Device in"=w5178) -> ("error out"=w5174:errorcluster, "State Machine.lvclass"=w5172:refnum<class "State Machine.lvclass">, "Device out"=w5177:refnum<class "Channel.lvclass">)  [unwired: 7 in]
            n2215 = call "Next State.vi"("error in (no error)"=w5174, "New_State"=12, "State Machine in"=w5172) -> ("error out"=w5173:errorcluster, "State Machine out"=w5171:refnum<class "State Machine.lvclass">)  [unwired: 7 in]
            n2216 = call-dynamic "Write State Machine.vi"("error in (no error)"=w5173, "State Machine.lvclass"=w5171, "Device in"=w5177) -> ("error out"=w5170:errorcluster, "Device out"=w5176:refnum<class "Channel.lvclass">)  [unwired: 7 in]
            n2217 = call-dynamic "Write Channel.vi"("error in (no error)"=w5170, "Channel.lvclass"=w5176, "Acquisition in"=w5194) -> ("error out"=w5192:errorcluster, "Acquisition out"=w5193:refnum<class "Acquisition.lvclass">)  [unwired: 7 in]
            n2218 = call-dynamic "Write AcquisitionA.vi"("error in (no error)"=w5192, "Acquisition.lvclass"=w5193, "S4ACS_GUI in"=w5195) -> ("error out"=w5190:errorcluster, "S4ACS_GUI out"=w5191:refnum<class "S4GUI.lvclass">)  [unwired: 7 in]
          }
          frame #1 {
            # "object"
            # "suffix"
            # "obsType"
            n2219 = call "Read AcquisitionB.vi"("error in (no error)"=w5248, "S4ACS_GUI in"=w5249) -> ("error out"=w5234:errorcluster, "Acquisition.lvclass"=w5235:refnum<class "Acquisition.lvclass">, "S4ACS_GUI out"=w5240:refnum<class "S4GUI.lvclass">)  [unwired: 7 in]
            n2220 = call-dynamic "Read Channel.vi"("error in (no error)"=w5234, "Acquisition in"=w5235) -> ("error out"=w5208:errorcluster, "Channel.lvclass"=w5210:refnum<class "Channel.lvclass">, "Acquisition out"=w5241:refnum<class "Acquisition.lvclass">)  [unwired: 7 in]
            n2221 = local read "Filter2"() -> (w5211:u8)
            n2222 = call-dynamic "Write Filter.vi"("error in (no error)"=w5208, "Filter"=w5211, "Channel in"=w5210) -> ("error out"=w5207:errorcluster, "Channel out"=w5209:refnum<class "Channel.lvclass">)  [unwired: 7 in]
            n2223 = call-dynamic "Read Interface.vi"("error in (no error)"=w5207, "Channel in"=w5209) -> ("error out"=w5222:errorcluster, "Interface.lvclass"=w5223:refnum<class "Interface.lvclass">, "Channel out"=w5236:refnum<class "Channel.lvclass">)  [unwired: 7 in]
            n2224 = call-dynamic "Write Suffix.vi"("error in (no error)"=w5222, "Suffix"=w5245, "Interface in"=w5223) -> ("error out"=w5231:errorcluster, "Interface out"=w5237:refnum<class "Interface.lvclass">)  [unwired: 7 in]
            n2225 = call-dynamic "Write ObsType.vi"("error in (no error)"=w5231, "ObsType"=w5230, "Interface in"=w5237) -> ("error out"=w5232:errorcluster, "Interface out"=w5238:refnum<class "Interface.lvclass">)  [unwired: 7 in]
            n2226 = call-dynamic "Write Object.vi"("error in (no error)"=w5232, "Object"=w5229, "Interface in"=w5238) -> ("error out"=w5233:errorcluster, "Interface out"=w5239:refnum<class "Interface.lvclass">)  [unwired: 7 in]
            n2227 = call-dynamic "Write Comments.vi"("error in (no error)"=w5233, "Comments"=w5244, "Interface in"=w5239) -> ("error out"=w5225:errorcluster, "Interface out"=w5224:refnum<class "Interface.lvclass">)  [unwired: 7 in]
            n2228 = call-dynamic "Write Observer.vi"("error in (no error)"=w5225, "Observer"=w5228, "Interface in"=w5224) -> ("error out"=w5226:errorcluster, "Interface out"=w5227:refnum<class "Interface.lvclass">)  [unwired: 7 in]
            n2229 = call-dynamic "Write Interface.vi"("error in (no error)"=w5226, "Interface.lvclass"=w5227, "Channel in"=w5236) -> ("error out"=w5215:errorcluster, "Channel out"=w5216:refnum<class "Channel.lvclass">)  [unwired: 7 in]
            n2230 = call-dynamic "Read State Machine.vi"("error in (no error)"=w5215, "Device in"=w5216) -> ("error out"=w5221:errorcluster, "State Machine.lvclass"=w5219:refnum<class "State Machine.lvclass">, "Device out"=w5214:refnum<class "Channel.lvclass">)  [unwired: 7 in]
            n2231 = call "Next State.vi"("error in (no error)"=w5221, "New_State"=12, "State Machine in"=w5219) -> ("error out"=w5220:errorcluster, "State Machine out"=w5218:refnum<class "State Machine.lvclass">)  [unwired: 7 in]
            n2232 = call-dynamic "Write State Machine.vi"("error in (no error)"=w5220, "State Machine.lvclass"=w5218, "Device in"=w5214) -> ("error out"=w5212:errorcluster, "Device out"=w5213:refnum<class "Channel.lvclass">)  [unwired: 7 in]
            n2233 = call-dynamic "Write Channel.vi"("error in (no error)"=w5212, "Channel.lvclass"=w5213, "Acquisition in"=w5241) -> ("error out"=w5243:errorcluster, "Acquisition out"=w5242:refnum<class "Acquisition.lvclass">)  [unwired: 7 in]
            n2234 = call "Write AcquisitionB.vi"("error in (no error)"=w5243, "Acquisition.lvclass"=w5242, "S4ACS_GUI in"=w5240) -> ("error out"=w5246:errorcluster, "S4ACS_GUI out"=w5247:refnum<class "S4GUI.lvclass">)  [unwired: 7 in]
          }
          frame #2 {
            # "object"
            # "suffix"
            # "obsType"
            n2235 = call-dynamic "Read AcquisitionC.vi"("error in (no error)"=w5291, "S4ACS_GUI in"=w5292) -> ("error out"=w5284:errorcluster, "Acquisition.lvclass"=w5283:refnum<class "Acquisition.lvclass">, "S4ACS_GUI out"=w5278:refnum<class "S4GUI.lvclass">)  [unwired: 7 in]
            n2236 = call-dynamic "Read Channel.vi"("error in (no error)"=w5284, "Acquisition in"=w5283) -> ("error out"=w5251:errorcluster, "Channel.lvclass"=w5253:refnum<class "Channel.lvclass">, "Acquisition out"=w5277:refnum<class "Acquisition.lvclass">)  [unwired: 7 in]
            n2237 = local read "Filter3"() -> (w5254:u8)
            n2238 = call-dynamic "Write Filter.vi"("error in (no error)"=w5251, "Filter"=w5254, "Channel in"=w5253) -> ("error out"=w5250:errorcluster, "Channel out"=w5252:refnum<class "Channel.lvclass">)  [unwired: 7 in]
            n2239 = call-dynamic "Read Interface.vi"("error in (no error)"=w5250, "Channel in"=w5252) -> ("error out"=w5269:errorcluster, "Interface.lvclass"=w5270:refnum<class "Interface.lvclass">, "Channel out"=w5282:refnum<class "Channel.lvclass">)  [unwired: 7 in]
            n2240 = call-dynamic "Write Suffix.vi"("error in (no error)"=w5269, "Suffix"=w5288, "Interface in"=w5270) -> ("error out"=w5287:errorcluster, "Interface out"=w5281:refnum<class "Interface.lvclass">)  [unwired: 7 in]
            n2241 = call-dynamic "Write ObsType.vi"("error in (no error)"=w5287, "ObsType"=w5273, "Interface in"=w5281) -> ("error out"=w5286:errorcluster, "Interface out"=w5280:refnum<class "Interface.lvclass">)  [unwired: 7 in]
            n2242 = call-dynamic "Write Object.vi"("error in (no error)"=w5286, "Object"=w5272, "Interface in"=w5280) -> ("error out"=w5285:errorcluster, "Interface out"=w5279:refnum<class "Interface.lvclass">)  [unwired: 7 in]
            n2243 = call-dynamic "Write Comments.vi"("error in (no error)"=w5285, "Comments"=w5274, "Interface in"=w5279) -> ("error out"=w5266:errorcluster, "Interface out"=w5265:refnum<class "Interface.lvclass">)  [unwired: 7 in]
            n2244 = call-dynamic "Write Observer.vi"("error in (no error)"=w5266, "Observer"=w5271, "Interface in"=w5265) -> ("error out"=w5267:errorcluster, "Interface out"=w5268:refnum<class "Interface.lvclass">)  [unwired: 7 in]
            n2245 = call-dynamic "Write Interface.vi"("error in (no error)"=w5267, "Interface.lvclass"=w5268, "Channel in"=w5282) -> ("error out"=w5260:errorcluster, "Channel out"=w5261:refnum<class "Channel.lvclass">)  [unwired: 7 in]
            n2246 = call-dynamic "Read State Machine.vi"("error in (no error)"=w5260, "Device in"=w5261) -> ("error out"=w5264:errorcluster, "State Machine.lvclass"=w5257:refnum<class "State Machine.lvclass">, "Device out"=w5259:refnum<class "Channel.lvclass">)  [unwired: 7 in]
            n2247 = call "Next State.vi"("error in (no error)"=w5264, "New_State"=12, "State Machine in"=w5257) -> ("error out"=w5263:errorcluster, "State Machine out"=w5256:refnum<class "State Machine.lvclass">)  [unwired: 7 in]
            n2248 = call-dynamic "Write State Machine.vi"("error in (no error)"=w5263, "State Machine.lvclass"=w5256, "Device in"=w5259) -> ("error out"=w5255:errorcluster, "Device out"=w5258:refnum<class "Channel.lvclass">)  [unwired: 7 in]
            n2249 = call-dynamic "Write Channel.vi"("error in (no error)"=w5255, "Channel.lvclass"=w5258, "Acquisition in"=w5277) -> ("error out"=w5275:errorcluster, "Acquisition out"=w5276:refnum<class "Acquisition.lvclass">)  [unwired: 7 in]
            n2250 = call-dynamic "Write AcquisitionC.vi"("error in (no error)"=w5275, "Acquisition.lvclass"=w5276, "S4ACS_GUI in"=w5278) -> ("error out"=w5289:errorcluster, "S4ACS_GUI out"=w5290:refnum<class "S4GUI.lvclass">)  [unwired: 7 in]
          }
          frame #3 {
            # "object"
            # "suffix"
            # "obsType"
            n2251 = call-dynamic "Read AcquisitionD.vi"("error in (no error)"=w5334, "S4ACS_GUI in"=w5335) -> ("error out"=w5327:errorcluster, "Acquisition.lvclass"=w5326:refnum<class "Acquisition.lvclass">, "S4ACS_GUI out"=w5321:refnum<class "S4GUI.lvclass">)  [unwired: 7 in]
            n2252 = call-dynamic "Read Channel.vi"("error in (no error)"=w5327, "Acquisition in"=w5326) -> ("error out"=w5294:errorcluster, "Channel.lvclass"=w5296:refnum<class "Channel.lvclass">, "Acquisition out"=w5320:refnum<class "Acquisition.lvclass">)  [unwired: 7 in]
            n2253 = local read "Filter4"() -> (w5297:u8)
            n2254 = call-dynamic "Write Filter.vi"("error in (no error)"=w5294, "Filter"=w5297, "Channel in"=w5296) -> ("error out"=w5293:errorcluster, "Channel out"=w5295:refnum<class "Channel.lvclass">)  [unwired: 7 in]
            n2255 = call-dynamic "Read Interface.vi"("error in (no error)"=w5293, "Channel in"=w5295) -> ("error out"=w5312:errorcluster, "Interface.lvclass"=w5313:refnum<class "Interface.lvclass">, "Channel out"=w5325:refnum<class "Channel.lvclass">)  [unwired: 7 in]
            n2256 = call-dynamic "Write Suffix.vi"("error in (no error)"=w5312, "Suffix"=w5331, "Interface in"=w5313) -> ("error out"=w5330:errorcluster, "Interface out"=w5324:refnum<class "Interface.lvclass">)  [unwired: 7 in]
            n2257 = call-dynamic "Write ObsType.vi"("error in (no error)"=w5330, "ObsType"=w5316, "Interface in"=w5324) -> ("error out"=w5329:errorcluster, "Interface out"=w5323:refnum<class "Interface.lvclass">)  [unwired: 7 in]
            n2258 = call-dynamic "Write Object.vi"("error in (no error)"=w5329, "Object"=w5315, "Interface in"=w5323) -> ("error out"=w5328:errorcluster, "Interface out"=w5322:refnum<class "Interface.lvclass">)  [unwired: 7 in]
            n2259 = call-dynamic "Write Comments.vi"("error in (no error)"=w5328, "Comments"=w5317, "Interface in"=w5322) -> ("error out"=w5311:errorcluster, "Interface out"=w5310:refnum<class "Interface.lvclass">)  [unwired: 7 in]
